vi "byte2nibbles.vi"(0 "byte":u8) -> (2 "high nibble":u8, 3 "low nibble":u8)   [LabVIEW 2014]
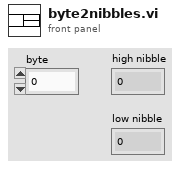
[diagram p1: front panel]
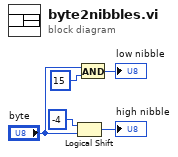
[diagram p0: block diagram]
diagram:
  n1 = Logical Shift(y=i16 -4, x="byte") -> (x << y=→"high nibble":u8)
  n2 = And(x="byte", y=u8 15) -> (x .and. y?=→"low nibble":u8)
